vi "Camera.vi"(8 "error in (no error) 2":cluster{"状态":bool, "代码":i32, "源":string} caption="错误输入（无错误）") -> (0 "error out (no error)":cluster{"状态":bool, "代码":i32, "源":string} caption="错误输入（无错误）")   [LabVIEW 2015, in "Debug.lvlib"]
uses:
  Debug.lvlib
  Support/Debug UI Refs.ctl
  <vilib>/vision/Image Controls.llb/IMAQ Image.ctl
  Support/Camera Configuration.ctl
  Sub VIs/CCD/Support/CCD Configuration.ctl
  <vilib>/userdefined/High Color/IMAQdx.ctl
  <vilib>/Utility/error.llb/Error Cluster From Error Code.vi
  <vilib>/ErrorRing/Error Ring.xnode
  support/Message Queue/Message Queue.lvlib
  support/User Event - Stop/User Event - Stop.lvlib
  Sub VIs/CCD/CCD.lvlib
panel:
  in  "退出":bool
  in  "停止按钮":bool
  in  "计算距离":bool
  in  "保存按钮":bool
  in  "开始":bool
  out "Image":T1(plugin-control)
  out "状态栏":string
  # "Camera Setting"
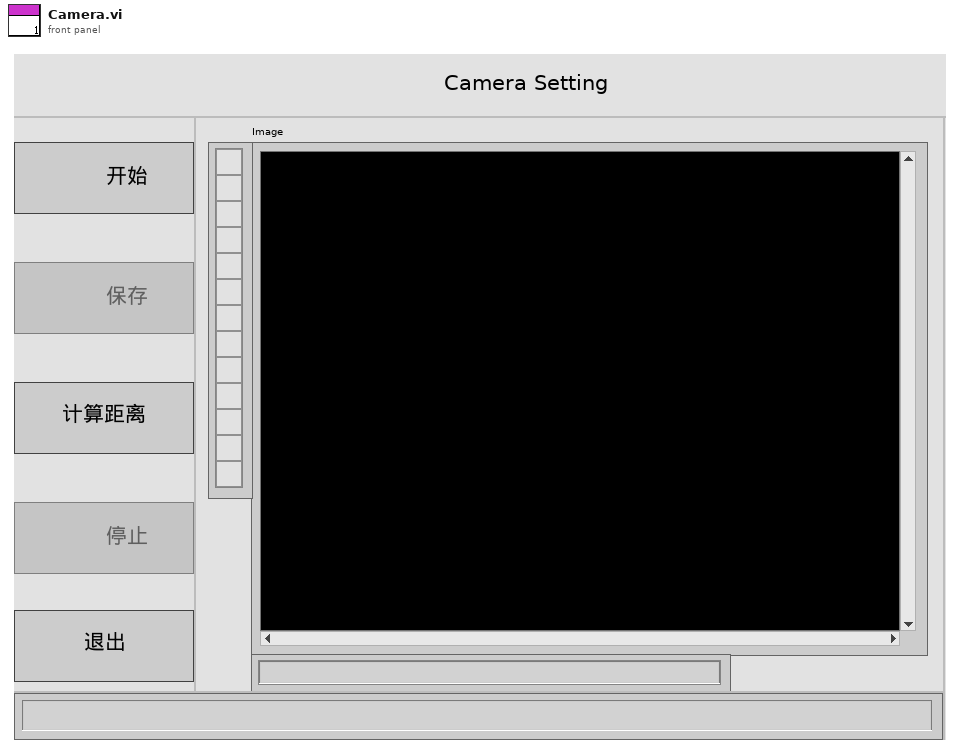
[diagram p1: front panel]
types:
  T1 = typedef "IMAQ Image.ctl" = refnum<image>
  T2 = typedef "Debug.lvlib/Camera Configuration.ctl" = cluster{"CCD Configuration":T3}
  T3 = typedef "CCD.lvlib/CCD Configuration.ctl" = cluster{"Session In":T4, "New Image":T1}
  T4 = typedef "IMAQdx.ctl" = refnum<k21>
  T5 = typedef "Debug.lvlib/Debug UI Refs.ctl" = cluster{"开始按钮引用句柄":refnum<vi>, "保持按钮引用句柄":refnum<vi>, "计算距离按钮l引用句柄":refnum<vi>, "停止按钮引用句柄":refnum<vi>, "状态栏引用句柄":refnum<vi>, "退出按钮引用句柄":refnum<vi>}
  T6 = typedef "Message Queue.lvlib/All Message Queues Camera.ctl" = cluster{"UI":refnum<queue>, "CAM":refnum<queue>, "Save":refnum<queue>}
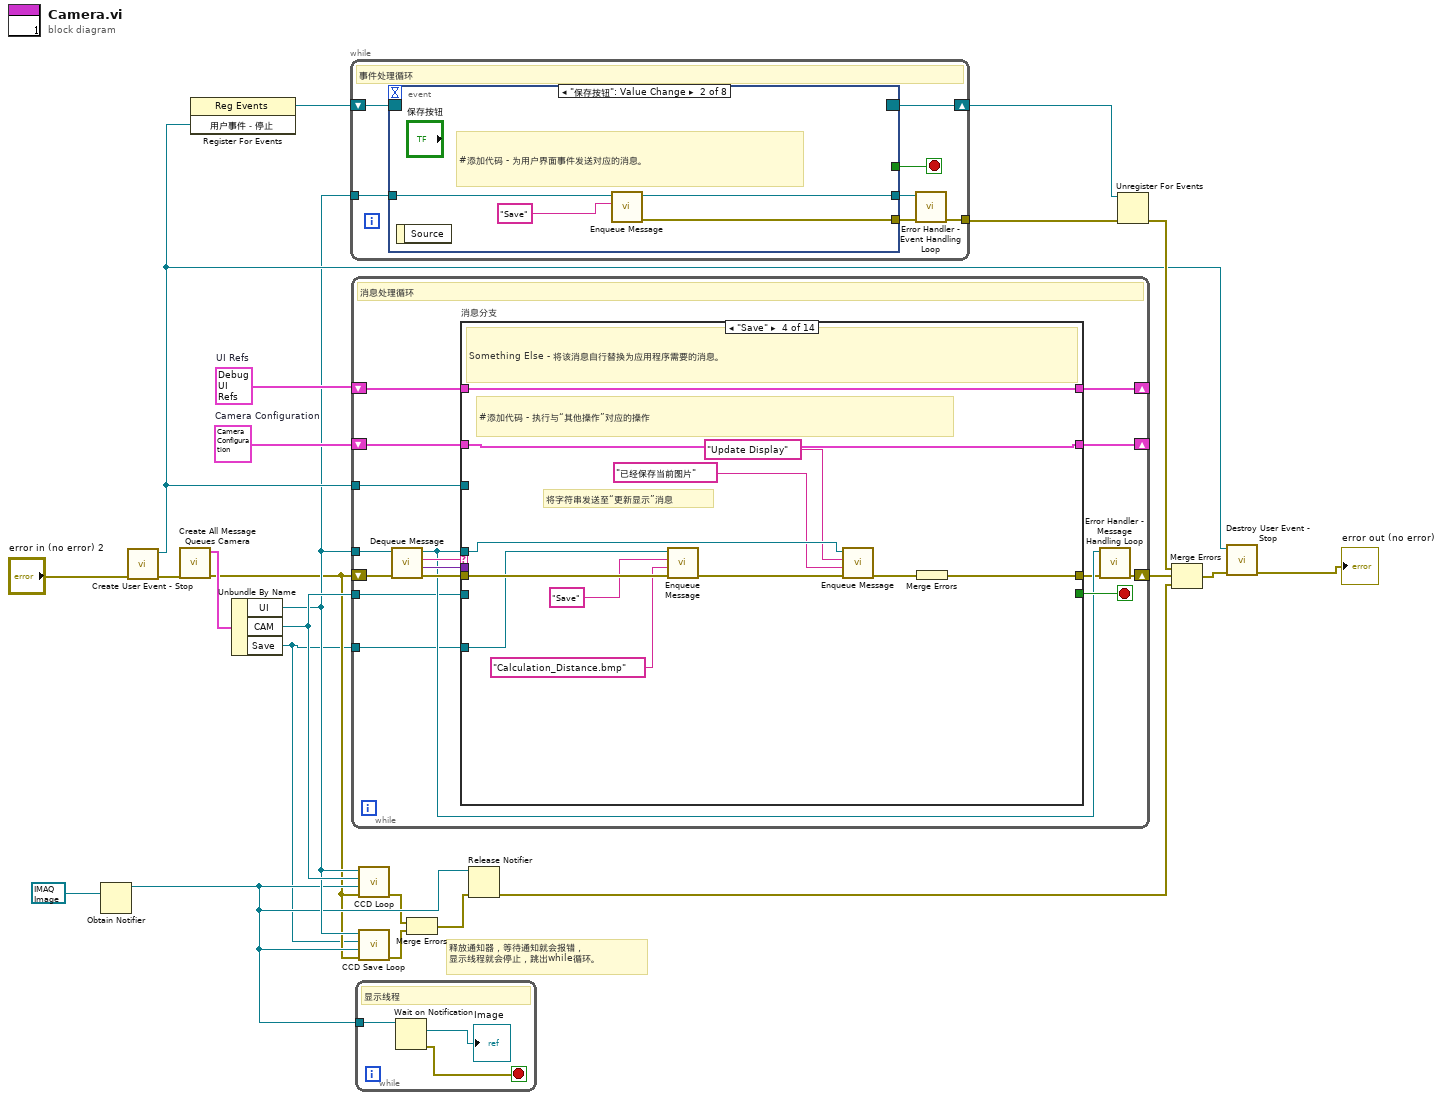
[diagram p0: block diagram]
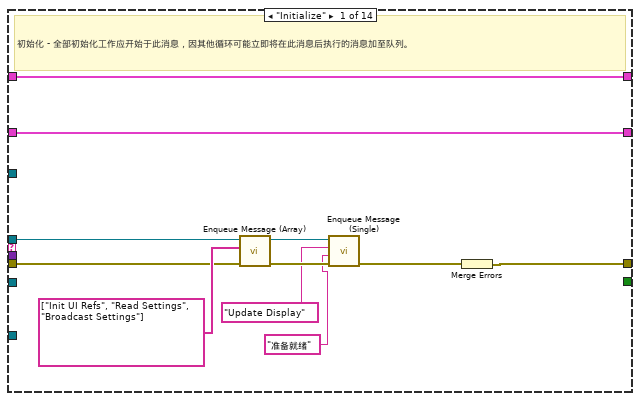
[diagram p2: hidden frame]
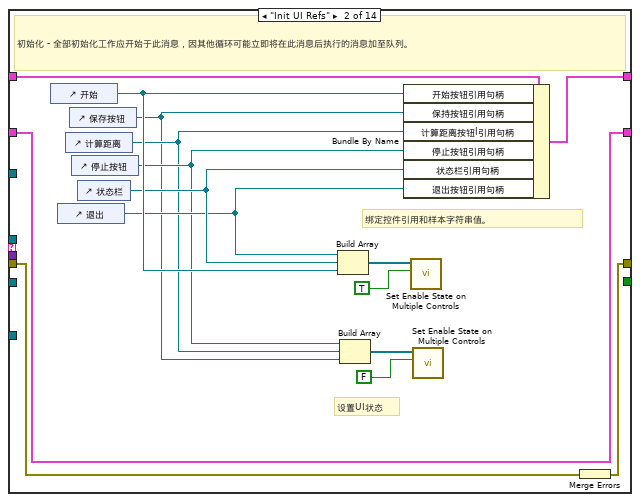
[diagram p3: hidden frame]
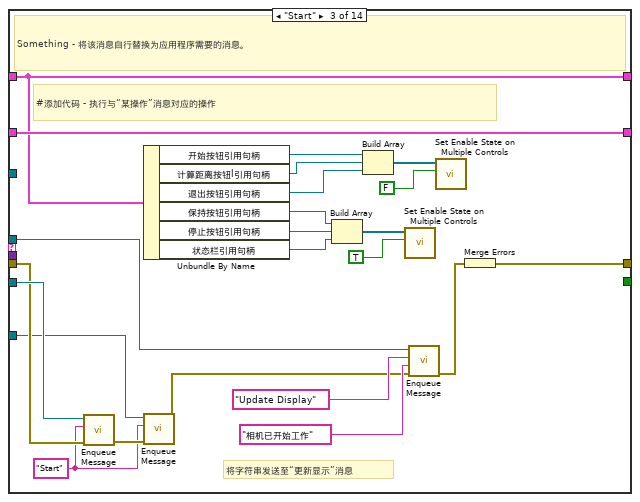
[diagram p4: hidden frame]
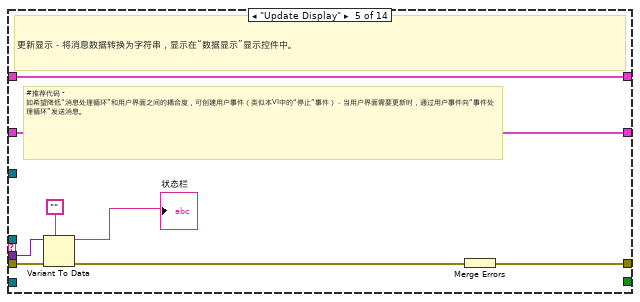
[diagram p5: hidden frame]
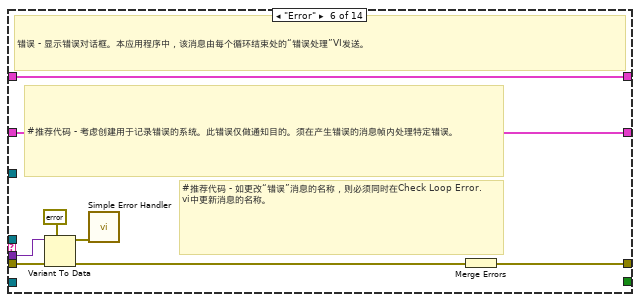
[diagram p6: hidden frame]
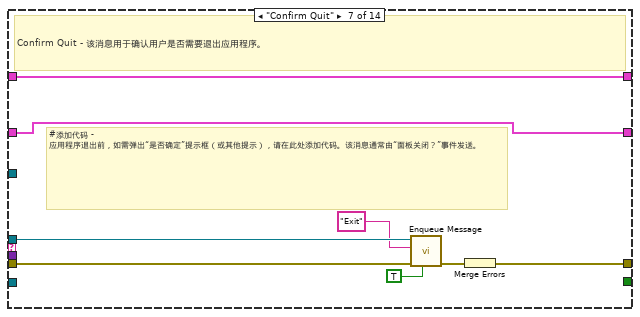
[diagram p7: hidden frame]
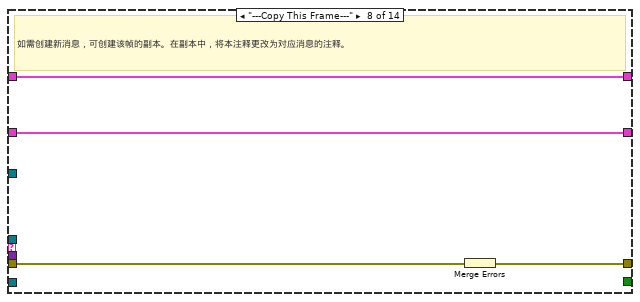
[diagram p8: hidden frame]
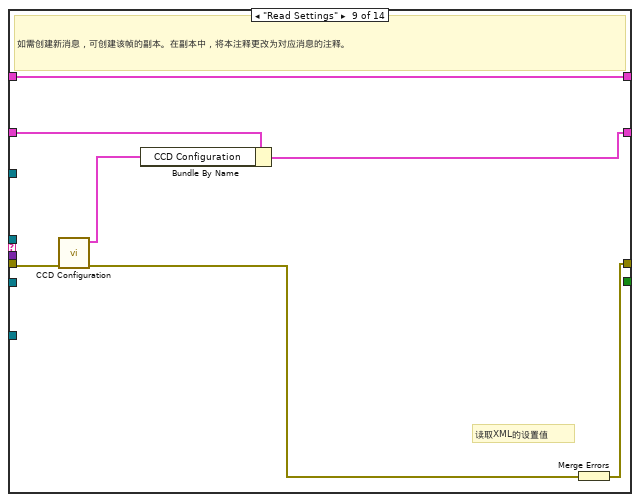
[diagram p9: hidden frame]
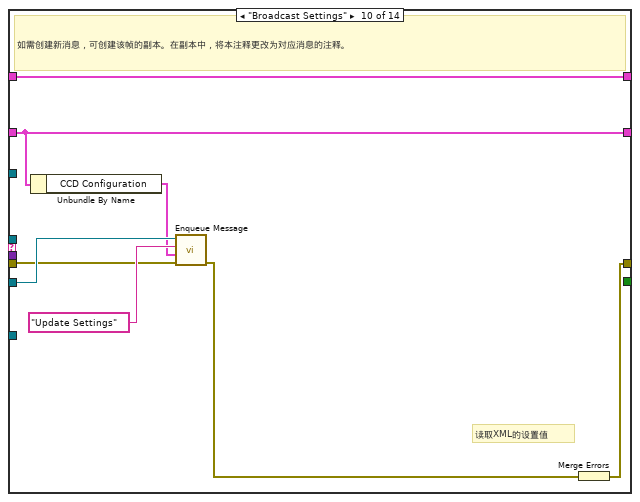
[diagram p10: hidden frame]
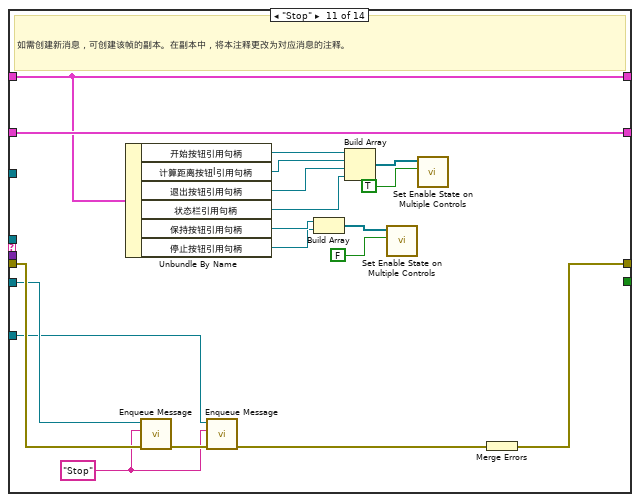
[diagram p11: hidden frame]
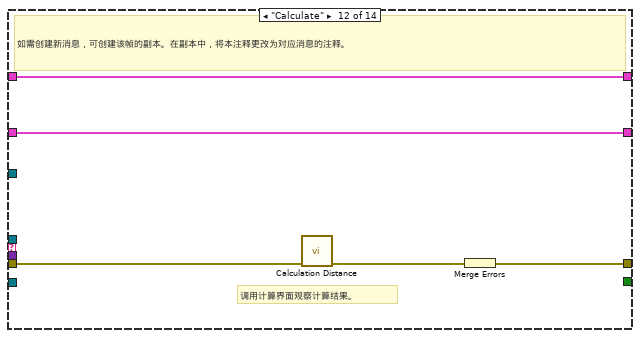
[diagram p12: hidden frame]
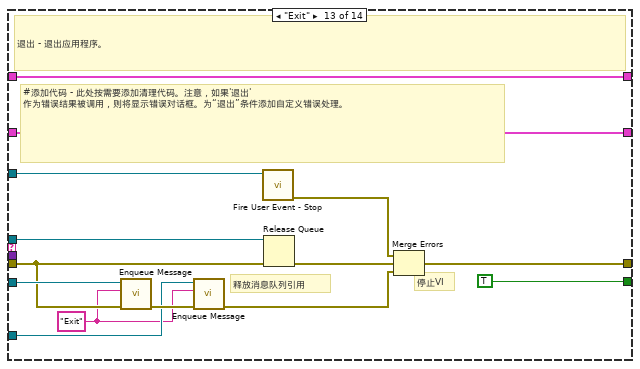
[diagram p13: hidden frame]
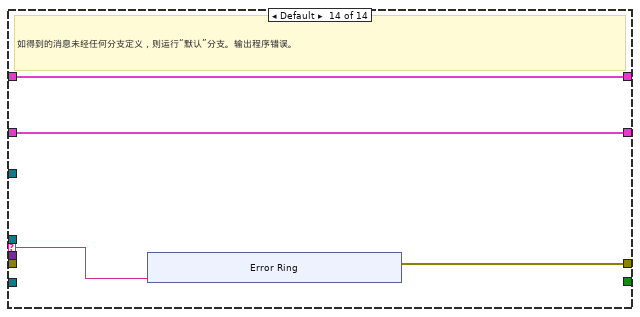
[diagram p14: hidden frame]
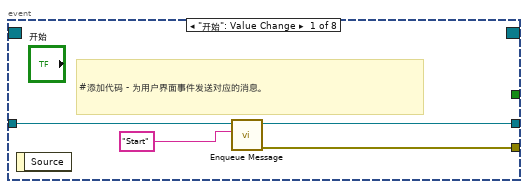
[diagram p15: hidden frame]
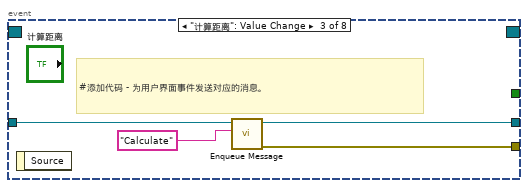
[diagram p16: hidden frame]
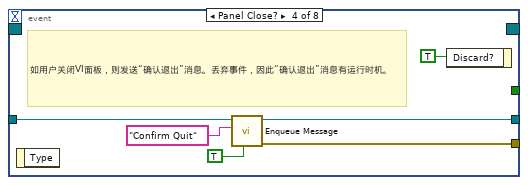
[diagram p17: hidden frame]
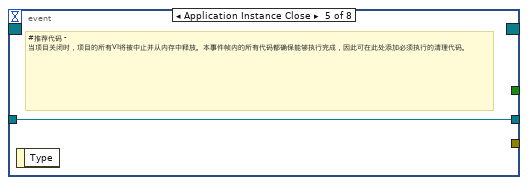
[diagram p18: hidden frame]
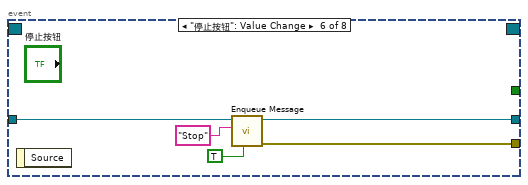
[diagram p19: hidden frame]
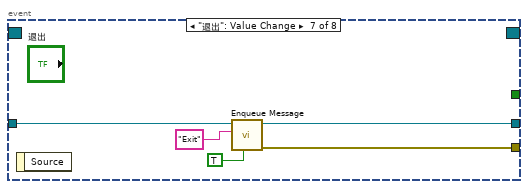
[diagram p20: hidden frame]
diagram:
  w10 = T2 {"CCD Configuration"={"Session In"="", "New Image"=refnum}}  # Camera Configuration
  w20 = T5 {"开始按钮引用句柄"=refnum, "保持按钮引用句柄"=refnum, "计算距离按钮l引用句柄"=refnum, "停止按钮引用句柄"=refnum, "状态栏引用句柄"=refnum, "退出按钮引用句柄"=refnum}  # UI Refs
  # "释放通知器，等待通知就会报错，\n显示线程就会停止，跳出while循环。"
  n1 = Obtain Notifier(notification data type=T1 refnum ("Image Out")) -> (notifier out=w6:refnum<notifier>)  [unwired: 3 in, 2 out]
  n2 = call "Create User Event - Stop.vi"("error in (no error)"="error in (no error) 2") -> ("error out"=w22:cluster{"状态":bool, "代码":i32, "源":string}, "用户事件－停止"=w15:refnum<user-event>)  [unwired: 9 in]
  n3 = call "Create All Message Queues Camera.vi"("error in (no error)"=w22) -> ("error out"=w5:cluster{"状态":bool, "代码":i32, "源":string}, "消息队列"=w23:T6)  [unwired: 9 in]
  n4 = register-events(w15) -> (reference out=w21:refnum<event-registration>)  [unwired: 2 in, 1 out]
  n5 = Unbundle By Name(w23) -> ("UI"=w7:refnum<queue>, "CAM"=w12:refnum<queue>, "Save"=w1:refnum<queue>)
  n6 = while {
    tunnel: w7 -> [w30]
    shift-right: [w28] -> w18
    shift-left: w21 -> [w29]
    tunnel: [w24] -> w19
    stop <- w26 stop-if-true
    # "事件处理循环"
    n7 = event shown="[1] \"保存按钮\": Value Change" {
      selector: w29 -> [_ _ _ _ _ _ _ _]
      dyn-events: [_ _ _ _ _ _ _ _] -> w28
      timeout: _ -> [_ _ _ _ _ _ _ _]
      tunnel: [_ _ _ _ _ _ _ TRUE ("Discard?")] -> w26
      tunnel: w30 -> [w34 w38 w42 w47 w49 w54 w59 w61]
      tunnel: [w31 w35 w39 w46 _ w53 w58 _] -> w27
      tunnel: [w33 w37 w41 w45 w49 w52 w57 w61] -> w25
      event "开始": Value Change {
        # "#添加代码 - 为用户界面事件发送对应的消息。"
        n8 = event-data() -> ()  [unwired: 1 in, 1 out]
        n9 = call-poly "Enqueue Message.vi"("消息"="Start" ("Message"), "消息队列"=w34) -> ("error out"=w31:cluster{"状态":bool, "代码":i32, "源":string}, "消息队列副本"=w33:refnum<queue>)  [unwired: 8 in]
      }
      event "保存按钮": Value Change {
        # "#添加代码 - 为用户界面事件发送对应的消息。"
        n10 = event-data() -> ()  [unwired: 1 in, 1 out]
        n11 = call-poly "Enqueue Message.vi"("消息"="Save" ("Message"), "消息队列"=w38) -> ("error out"=w35:cluster{"状态":bool, "代码":i32, "源":string}, "消息队列副本"=w37:refnum<queue>)  [unwired: 8 in]
      }
      event "计算距离": Value Change {
        # "#添加代码 - 为用户界面事件发送对应的消息。"
        n12 = event-data() -> ()  [unwired: 1 in, 1 out]
        n13 = call-poly "Enqueue Message.vi"("消息"="Calculate" ("Message"), "消息队列"=w42) -> ("error out"=w39:cluster{"状态":bool, "代码":i32, "源":string}, "消息队列副本"=w41:refnum<queue>)  [unwired: 8 in]
      }
      event Panel Close? {
        # "如用户关闭VI面板，则发送“确认退出”消息。丢弃事件，因此“确认退出”消息有运行时机。"
        n14 = event-data() -> ()  [unwired: 1 in, 1 out]
        n15 = call-poly "Enqueue Message.vi"("优先消息？ (F)"=TRUE ("Priority Message? (F)"), "消息"="Confirm Quit" ("Message"), "消息队列"=w47) -> ("error out"=w46:cluster{"状态":bool, "代码":i32, "源":string}, "消息队列副本"=w45:refnum<queue>)  [unwired: 7 in]
        n16 = event-data ("Event Filter Node")("Discard?"=TRUE) -> ()  [unwired: 1 in, 1 out]
      }
      event Application Instance Close {
        # "#推荐代码 - 当项目关闭时，项目的所有VI将被中止并从内存中释放。本事件帧内的所有代码都确保能够执行完成，因此可在此处添加必须执行的清理代码。"
        n17 = event-data() -> ()  [unwired: 1 in, 1 out]
      }
      event "停止按钮": Value Change {
        n18 = event-data() -> ()  [unwired: 1 in, 1 out]
        n19 = call-poly "Enqueue Message.vi"("优先消息？ (F)"=TRUE ("Priority Message? (F)"), "消息"="Stop" ("Message"), "消息队列"=w54) -> ("error out"=w53:cluster{"状态":bool, "代码":i32, "源":string}, "消息队列副本"=w52:refnum<queue>)  [unwired: 7 in]
      }
      event "退出": Value Change {
        n20 = event-data() -> ()  [unwired: 1 in, 1 out]
        n21 = call-poly "Enqueue Message.vi"("优先消息？ (F)"=TRUE ("Priority Message? (F)"), "消息"="Exit" ("Message"), "消息队列"=w59) -> ("error out"=w58:cluster{"状态":bool, "代码":i32, "源":string}, "消息队列副本"=w57:refnum<queue>)  [unwired: 7 in]
      }
      event User Event {
        (unwired) "“退出”按钮按下" ("VI Stopped")
        # "消息处理循环对“退出”消息进行处理，触发该事件，从而使事件处理循环停止运行。"
        n22 = event-data() -> ()  [unwired: 1 in, 1 out]
      }
    }
    n23 = call "Error Handler - Event Handling Loop.vi"("error in (no error)"=w27, "消息队列"=w25) -> ("错误输入副本"=w24:cluster{"状态":bool, "代码":i32, "源":string})  [unwired: 8 in, 1 out]
  }
  n24 = while {
    tunnel: w7 -> [w69]
    shift-right: [w76] -> _
    shift-left: w20 -> [w77]
    tunnel: w15 -> [w74]
    tunnel: w12 -> [w66]
    shift-right: [w64] -> _
    shift-left: w10 -> [w65]
    shift-right: [w63] -> w9
    shift-left: w5 -> [w73]
    tunnel: w1 -> [w62]
    stop <- w75 stop-if-true
    # "消息处理循环"
    n25 = call "Dequeue Message.vi"("error in (no error)"=w73, "消息队列"=w69) -> ("error out"=w72:cluster{"状态":bool, "代码":i32, "源":string}, "消息数据"=w70:variant, "消息"=w71:string, "消息队列副本"=w68:refnum<queue>)  [unwired: 6 in]
    n26 = case "消息分支" shown="\"Save\"" w71 {
      selector: w71 -> [_ _ _ _ _ _ _ _ _ _ _ _ _ w221]
      tunnel: w68 -> [w85 _ w125 w135 _ _ w158 _ _ _ _ _ w219 _]
      tunnel: w72 -> [w83 w90 w121 w131 w144 w154 w162 w166 w171 w176 w199 w202 w211 _]
      tunnel: [w88 w103 w126 w137 w145 w148 w160 w164 w172 w180 w200 w204 w215 w222] -> w67
      tunnel: w77 -> [w87 w102 w118 w138 w146 w153 w161 w165 w173 w181 w189 w205 w218 w223]
      tunnel: [w87 w101 w118 w138 w146 w153 w161 w165 w173 w181 w189 w205 w218 w223] -> w76
      tunnel: [_ _ _ _ _ _ _ _ _ _ _ _ TRUE _] -> w75
      tunnel: w70 -> [_ _ _ _ w143 w152 _ _ _ _ _ _ _ _]
      tunnel: w74 -> [_ _ _ _ _ _ _ _ _ _ _ _ w214 _]
      tunnel: w66 -> [_ _ w122 _ _ _ _ _ _ w179 w198 _ w212 _]
      tunnel: w65 -> [w86 w89 w119 w132 w139 w147 w155 w163 w169 w174 w190 w203 w210 w220]
      tunnel: [w86 w89 w119 w132 w139 w147 w155 w163 w167 w174 w190 w203 w210 w220] -> w64
      tunnel: w62 -> [_ _ w105 w129 _ _ _ _ _ _ w183 _ w207 _]
      frame "Initialize" {
        # "初始化 - 全部初始化工作应开始于此消息，因其他循环可能立即将在此消息后执行的消息加至队列。"
        n27 = call "Enqueue Message (Array).vi"("error in (no error)"=w83, "消息数组"=string[] ["Init UI Refs", "Read Settings", "Broadcast Settings"], "消息队列"=w85) -> ("error out"=w82:cluster{"状态":bool, "代码":i32, "源":string}, "消息队列副本"=w80:refnum<queue>)  [unwired: 7 in]
        n28 = call "Enqueue Message (Single).vi"("error in (no error)"=w82, "消息数据"="准备就绪" ("消息"), "消息"="Update Display", "消息队列"=w80) -> ("error out"=w81:cluster{"状态":bool, "代码":i32, "源":string})  [unwired: 6 in, 1 out]
        n29 = Merge Errors(w81) -> (w88:errorcluster)
      }
      frame "Init UI Refs" {
        # "设置UI状态"
        # "绑定控件引用和样本字符串值。"
        # "初始化 - 全部初始化工作应开始于此消息，因其他循环可能立即将在此消息后执行的消息加至队列。"
        n30 = control-ref of="开始"() -> (w100:refnum<vi>)
        n31 = control-ref of="退出"() -> (w98:refnum<vi>)
        n32 = control-ref of="计算距离"() -> (w92:refnum<vi>)
        n33 = control-ref of="保存按钮"() -> (w91:refnum<vi>)
        n34 = control-ref of="停止按钮"() -> (w93:refnum<vi>)
        n35 = control-ref of="状态栏"() -> (w99:refnum<vi>)
        n36 = Build Array(w98, w99, w100) -> (w97:refnum<vi>[])
        n37 = Build Array(w93, w92, w91) -> (w95:refnum<vi>[])
        n38 = Bundle By Name(cluster=w102, "开始按钮引用句柄"=w100, "保持按钮引用句柄"=w91, "计算距离按钮l引用句柄"=w92, "停止按钮引用句柄"=w93, "状态栏引用句柄"=w99, "退出按钮引用句柄"=w98) -> (w101:T5)
        n39 = call "Set Enable State on Multiple Controls.vi"("启用？"=TRUE, "控件"=w97) -> ()  [unwired: 10 in]
        n40 = call "Set Enable State on Multiple Controls.vi"("启用？"=FALSE, "控件"=w95) -> ()  [unwired: 10 in]
        n41 = Merge Errors(w90) -> (w103:errorcluster)
      }
      frame "Start" {
        w104 = "Start" ("消息")
        # "将字符串发送至“更新显示”消息"
        # "#添加代码 - 执行与“某操作”消息对应的操作"
        # "Something - 将该消息自行替换为应用程序需要的消息。"
        n42 = call-poly "Enqueue Message.vi"("error in (no error)"=w121, "消息"=w104, "消息队列"=w122) -> ("error out"=w107:cluster{"状态":bool, "代码":i32, "源":string})  [unwired: 7 in, 1 out]
        n43 = Unbundle By Name(w118) -> ("开始按钮引用句柄"=w115:refnum<vi>, "计算距离按钮l引用句柄"=w114:refnum<vi>, "退出按钮引用句柄"=w113:refnum<vi>, "保持按钮引用句柄"=w110:refnum<vi>, "停止按钮引用句柄"=w109:refnum<vi>, "状态栏引用句柄"=w108:refnum<vi>)
        n44 = call-poly "Enqueue Message.vi"("error in (no error)"=w107, "消息"=w104, "消息队列"=w105) -> ("error out"=w106:cluster{"状态":bool, "代码":i32, "源":string})  [unwired: 7 in, 1 out]
        n45 = Build Array(w110, w109, w108) -> (w112:refnum<vi>[])
        n46 = Build Array(w115, w114, w113) -> (w117:refnum<vi>[])
        n47 = call "Set Enable State on Multiple Controls.vi"("启用？"=TRUE, "控件"=w112) -> ()  [unwired: 10 in]
        n48 = call-poly "Enqueue Message.vi"("error in (no error)"=w106, "消息数据"="相机已开始工作" ("\"Do Something\" button pressed"), "消息"="Update Display" ("Message"), "消息队列"=w125) -> ("error out"=w120:cluster{"状态":bool, "代码":i32, "源":string})  [unwired: 6 in, 1 out]
        n49 = call "Set Enable State on Multiple Controls.vi"("启用？"=FALSE, "控件"=w117) -> ()  [unwired: 10 in]
        n50 = Merge Errors(w120) -> (w126:errorcluster)
      }
      frame "Save" {
        # "将字符串发送至“更新显示”消息"
        # "#添加代码 - 执行与“其他操作”对应的操作"
        # "Something Else - 将该消息自行替换为应用程序需要的消息。"
        n51 = call-poly "Enqueue Message.vi"("error in (no error)"=w131, "消息数据"="Calculation_Distance.bmp" ("消息"), "消息"="Save", "消息队列"=w129) -> ("error out"=w130:cluster{"状态":bool, "代码":i32, "源":string})  [unwired: 6 in, 1 out]
        n52 = call-poly "Enqueue Message.vi"("error in (no error)"=w130, "消息数据"="已经保存当前图片" ("\"Do Something Else\" button pressed"), "消息"="Update Display" ("Message"), "消息队列"=w135) -> ("error out"=w136:cluster{"状态":bool, "代码":i32, "源":string})  [unwired: 6 in, 1 out]
        n53 = Merge Errors(w136) -> (w137:errorcluster)
      }
      frame "Update Display" {
        # "#推荐代码 - 如希望降低“消息处理循环”和用户界面之间的耦合度，可创建用户事件（类似本VI中的“停止”事件）－当用户界面需要更新时，通过用户事件向“事件处理循环”发送消息。"
        # "更新显示－将消息数据转换为字符串，显示在“数据显示”显示控件中。"
        n54 = Variant To Data(error in=w144, type="", Variant=w143) -> (data=→"状态栏":string, error out=w141:errorcluster)
        n55 = Merge Errors(w141) -> (w145:errorcluster)
      }
      frame "Error" {
        # "#推荐代码 - 如更改“错误”消息的名称，则必须同时在Check Loop Error.vi中更新消息的名称。"
        # "#推荐代码 - 考虑创建用于记录错误的系统。此错误仅做通知目的。须在产生错误的消息帧内处理特定错误。"
        # "错误 - 显示错误对话框。本应用程序中，该消息由每个循环结束处的“错误处理”VI发送。"
        n56 = Variant To Data(error in=w154, type=errorcluster {"status"=FALSE, "code"=0, "source"=""} ("error constant"), Variant=w152) -> (data=w150:errorcluster, error out=w149:errorcluster)
        n57 = call <vilib>:"Simple Error Handler.vi"("error in (no error)"=w150) -> ()  [unwired: 4 in, 5 out]
        n58 = Merge Errors(w149) -> (w148:errorcluster)
      }
      frame "Confirm Quit" {
        # "#添加代码 - 应用程序退出前，如需弹出“是否确定”提示框（或其他提示），请在此处添加代码。该消息通常由“面板关闭？”事件发送。"
        # "Confirm Quit - 该消息用于确认用户是否需要退出应用程序。"
        n59 = call-poly "Enqueue Message.vi"("优先消息？ (F)"=TRUE ("Priority Message? (F)"), "error in (no error)"=w162, "消息"="Exit" ("Message"), "消息队列"=w158) -> ("error out"=w159:cluster{"状态":bool, "代码":i32, "源":string})  [unwired: 6 in, 1 out]
        n60 = Merge Errors(w159) -> (w160:errorcluster)
      }
      frame "---Copy This Frame---" {
        # "如需创建新消息，可创建该帧的副本。在副本中，将本注释更改为对应消息的注释。"
        n61 = Merge Errors(w166) -> (w164:errorcluster)
      }
      frame "Read Settings" {
        # "读取XML的设置值"
        # "如需创建新消息，可创建该帧的副本。在副本中，将本注释更改为对应消息的注释。"
        n62 = call "CCD Configuration.vi"("error in (no error)"=w171) -> ("error out"=w170:errorcluster, "CCD Configuration"=w168:T3)  [unwired: 9 in]
        n63 = Bundle By Name(cluster=w169, "CCD Configuration"=w168) -> (w167:T2)
        n64 = Merge Errors(w170) -> (w172:errorcluster)
      }
      frame "Broadcast Settings" {
        # "读取XML的设置值"
        # "如需创建新消息，可创建该帧的副本。在副本中，将本注释更改为对应消息的注释。"
        n65 = Unbundle By Name(w174) -> ("CCD Configuration"=w177:T3)
        n66 = call-poly "Enqueue Message.vi"("error in (no error)"=w176, "消息数据"=w177, "消息"="Update Settings", "消息队列"=w179) -> ("error out"=w175:cluster{"状态":bool, "代码":i32, "源":string})  [unwired: 6 in, 1 out]
        n67 = Merge Errors(w175) -> (w180:errorcluster)
      }
      frame "Stop" {
        w182 = "Stop" ("消息")
        # "如需创建新消息，可创建该帧的副本。在副本中，将本注释更改为对应消息的注释。"
        n68 = Unbundle By Name(w189) -> ("开始按钮引用句柄"=w195:refnum<vi>, "计算距离按钮l引用句柄"=w194:refnum<vi>, "退出按钮引用句柄"=w193:refnum<vi>, "状态栏引用句柄"=w186:refnum<vi>, "保持按钮引用句柄"=w188:refnum<vi>, "停止按钮引用句柄"=w187:refnum<vi>)
        n69 = call-poly "Enqueue Message.vi"("error in (no error)"=w199, "消息"=w182, "消息队列"=w198) -> ("error out"=w185:cluster{"状态":bool, "代码":i32, "源":string})  [unwired: 7 in, 1 out]
        n70 = call-poly "Enqueue Message.vi"("error in (no error)"=w185, "消息"=w182, "消息队列"=w183) -> ("error out"=w184:cluster{"状态":bool, "代码":i32, "源":string})  [unwired: 7 in, 1 out]
        n71 = Build Array(w188, w187) -> (w192:refnum<vi>[])
        n72 = Build Array(w195, w194, w193, w186) -> (w197:refnum<vi>[])
        n73 = call "Set Enable State on Multiple Controls.vi"("启用？"=FALSE, "控件"=w192) -> ()  [unwired: 10 in]
        n74 = call "Set Enable State on Multiple Controls.vi"("启用？"=TRUE, "控件"=w197) -> ()  [unwired: 10 in]
        n75 = Merge Errors(w184) -> (w200:errorcluster)
      }
      frame "Calculate" {
        # "调用计算界面观察计算结果。"
        # "如需创建新消息，可创建该帧的副本。在副本中，将本注释更改为对应消息的注释。"
        n76 = call "Calculation Distance.vi"("error in"=w202) -> ("error out"=w201:errorcluster)  [unwired: 10 in]
        n77 = Merge Errors(w201) -> (w204:errorcluster)
      }
      frame "Exit" {
        w206 = "Exit" ("消息")
        # "停止VI"
        # "释放消息队列引用"
        # "#添加代码 - 此处按需要添加清理代码。注意，如果'退出' 作为错误结果被调用，则将显示错误对话框。为“退出”条件添加自定义错误处理。"
        # "退出 - 退出应用程序。"
        n78 = call-poly "Enqueue Message.vi"("error in (no error)"=w211, "消息"=w206, "消息队列"=w212) -> ("error out"=w209:cluster{"状态":bool, "代码":i32, "源":string})  [unwired: 7 in, 1 out]
        n79 = call-poly "Enqueue Message.vi"("error in (no error)"=w209, "消息"=w206, "消息队列"=w207) -> ("error out"=w208:cluster{"状态":bool, "代码":i32, "源":string})  [unwired: 7 in, 1 out]
        n80 = call "Fire User Event - Stop.vi"("用户事件－停止"=w214) -> ("error out"=w213:cluster{"状态":bool, "代码":i32, "源":string})  [unwired: 10 in]
        n81 = Release Queue(queue=w219, error in (no error)=w211) -> (error out=w216:errorcluster)  [unwired: 1 in, 2 out]
        n82 = Merge Errors(w213, w216, w208) -> (w215:errorcluster)
      }
      frame Default {
        # "如得到的消息未经任何分支定义，则运行“默认”分支。输出程序错误。"
        n83 = xnode ("Error Ring")("parameter 0"=w221) -> ("error out"=w222:errorcluster)
      }
    }
    n84 = call "Error Handler - Message Handling Loop.vi"("error in (no error)"=w67, "消息队列"=w68) -> ("错误输入副本"=w63:cluster{"状态":bool, "代码":i32, "源":string})  [unwired: 8 in, 1 out]
  }
  n85 = while {
    tunnel: w6 -> [w233]
    stop <- w231 stop-if-true
    # "显示线程"
    n86 = Wait on Notification(notifier=w233) -> (notification=→"Image":T1, error out=w231:errorcluster)  [unwired: 3 in, 2 out]
  }
  n87 = call "CCD Loop.vi"("error in (no error)"=w5, "数据通知器"=w6, "CAM"=w12, "Director"=w7) -> ("error out"=w4:errorcluster)  [unwired: 7 in]
  n88 = call "CCD Save Loop.vi"("error in (no error)"=w5, "数据通知器"=w6, "Save"=w1, "Director"=w7) -> ("error out"=w3:cluster{"状态":bool, "代码":i32, "源":string})  [unwired: 7 in]
  n89 = Merge Errors(w4, w3) -> (w2:errorcluster)
  n90 = Release Notifier(notifier=w6, error in (no error)=w2) -> (error out=w8:errorcluster)  [unwired: 1 in, 2 out]
  n91 = Unregister For Events(event registration refnum=w18, error in=w19) -> (error out=w17:errorcluster)
  n92 = Merge Errors(w17, w9, w8) -> (w16:errorcluster)
  n93 = call "Destroy User Event - Stop.vi"("error in (no error)"=w16, "用户事件－停止"=w15) -> ("error out"=→"error out (no error)":cluster{"状态":bool, "代码":i32, "源":string})  [unwired: 9 in]
